vi "DistanceBallToTarget.vi"(8 "error in (no error)":errorcluster, 9 "Target":dbl[](array[numeric]), 10 "Ball":refnum<class "Ball.lvclass">, 11 "Utilities in":refnum<class "Utilities.lvclass">) -> (0 "error out":errorcluster, 2 "Distance Ball To Target":dbl, 3 "Utilities out":refnum<class "Utilities.lvclass">)   [LabVIEW 2023, in "Utilities.lvclass"]
uses:
  Utilities.lvclass
  Ball_class/Ball.lvclass
  Object_class/Object.lvclass/Object.ctl
  Object_class/Read x.vi
  Object_class/Read y.vi
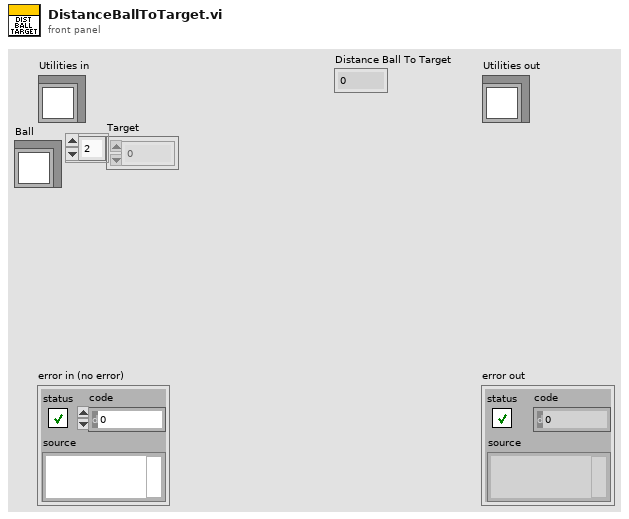
[diagram p1: front panel]
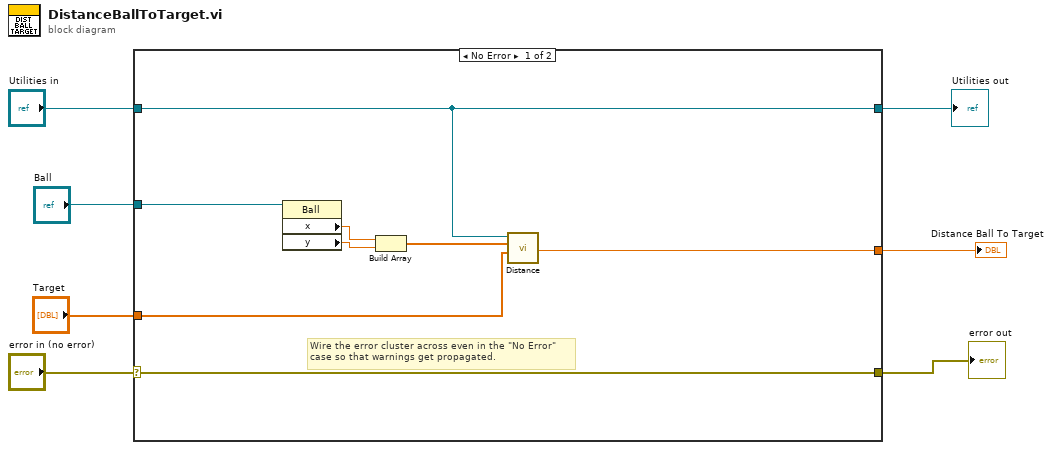
[diagram p0: block diagram]
diagram:
  n1 = case shown="No Error" "error in (no error)" {
    selector: "error in (no error)" -> [w15 w17]
    tunnel: [w15 w17] -> w6
    tunnel: [w11 w16] -> w4
    tunnel: "Utilities in" -> [w11 w16]
    tunnel: "Ball" -> [w10 _]
    tunnel: "Target" -> [w9 _]
    tunnel: [w8 _] -> w1
    frame No Error {
      # "Wire the error cluster across even in the \"No Error\"\ncase so that warnings get propagated."
      n2 = property class="Ball"(reference=w10) -> ("x"=w14:dbl, "y"=w13:dbl)  [unwired: 1 in, 2 out]
      n3 = Build Array(w14, w13) -> (w12:dbl[])
      n4 = call "Distance.vi"("P1"=w9, "P2"=w12, "Utilities in"=w11) -> ("Distance"=w8:dbl)  [unwired: 6 in, 2 out]
    }
    frame Error {
    }
  }
  "error out" <- w6
  "Utilities out" <- w4
  "Distance Ball To Target" <- w1
